vi "Garbagio-AB_BC_Chopper.vi"(9 "Portion of data":cluster{dbl, dbl}(slide)={0.75, 0.25} scale=0.0..1.0, 10 "Array of Clusters BC":cluster{dbl[], dbl[]}[](array[cluster]), 11 "Array of Clusters AB":cluster{dbl[], dbl[]}[](array[cluster])) -> (2 "Chopped AB thing":cluster{dbl[], dbl[]}, 3 "Chopped BC thing":cluster{dbl[], dbl[]})   [LabVIEW 2016]
uses:
  <vilib>/Analysis/2dsp.llb/Decimate (single shot, DBL).vi
  <vilib>/Analysis/NI_AALPro.lvlib
panel:
  in  "Decimate point":dbl=1e-10 format="%#_1f"
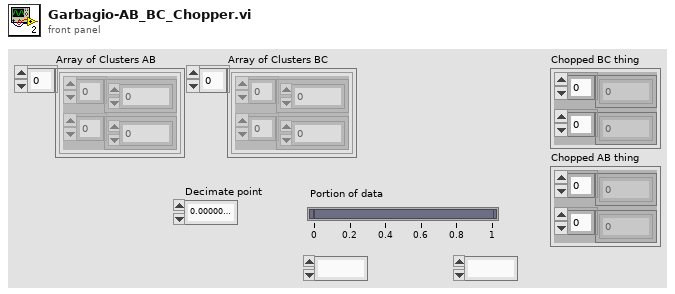
[diagram p1: front panel]
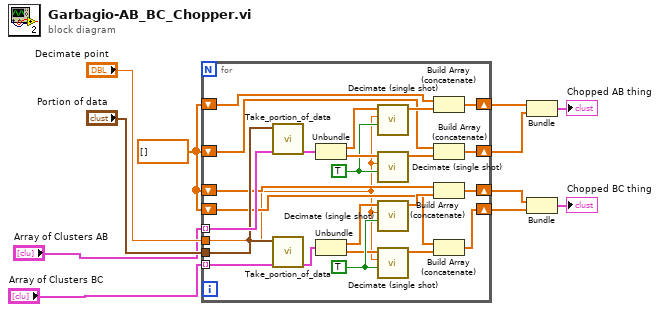
[diagram p0: block diagram]
diagram:
  w7 = dbl[] []
  n1 = for {
    tunnel: "Array of Clusters AB" -> [w35] mode=indexing
    tunnel: "Array of Clusters BC" -> [w18] mode=indexing
    tunnel: "Portion of data" -> [w17]
    tunnel: "Decimate point" -> [w12]
    shift-right: [w30] -> w9
    shift-left: w7 -> [w28]
    shift-right: [w26] -> w8
    shift-left: w7 -> [w25]
    shift-right: [w16] -> w6
    shift-left: w7 -> [w15]
    shift-right: [w14] -> w5
    shift-left: w7 -> [w13]
    w21 = TRUE ("averaging")
    w32 = TRUE ("averaging")
    n2 = call <userlib>:"Take_portion_of_data.vi"("input IV"=w35, "Slide"=w17) -> ("Output IV"=w31:cluster{dbl[], dbl[]})  [unwired: 5 in]
    n3 = call <userlib>:"Take_portion_of_data.vi"("input IV"=w18, "Slide"=w17) -> ("Output IV"=w22:cluster{dbl[], dbl[]})  [unwired: 5 in]
    n4 = Unbundle(w31) -> (w33:dbl[], w34:dbl[])
    n5 = Unbundle(w22) -> (w20:dbl[], w19:dbl[])
    n6 = call-poly <vilib>:"Decimate (single shot).vi"("averaging"=w32, "decimating factor"=w12, "X"=w33) -> ("Decimated Array"=w29:dbl[])  [unwired: 7 in, 1 out]
    n7 = call-poly <vilib>:"Decimate (single shot).vi"("averaging"=w32, "decimating factor"=w12, "X"=w34) -> ("Decimated Array"=w27:dbl[])  [unwired: 7 in, 1 out]
    n8 = call-poly <vilib>:"Decimate (single shot).vi"("averaging"=w21, "decimating factor"=w12, "X"=w20) -> ("Decimated Array"=w23:dbl[])  [unwired: 7 in, 1 out]
    n9 = call-poly <vilib>:"Decimate (single shot).vi"("averaging"=w21, "decimating factor"=w12, "X"=w19) -> ("Decimated Array"=w24:dbl[])  [unwired: 7 in, 1 out]
    n10 = Build Array (concatenate)(w28, w29) -> (w30:dbl[])
    n11 = Build Array (concatenate)(w25, w27) -> (w26:dbl[])
    n12 = Build Array (concatenate)(w15, w23) -> (w16:dbl[])
    n13 = Build Array (concatenate)(w13, w24) -> (w14:dbl[])
  }
  n14 = Bundle(w9, w8) -> (→"Chopped AB thing":cluster{dbl[], dbl[]})  [unwired: 1 in]
  n15 = Bundle(w6, w5) -> (→"Chopped BC thing":cluster{dbl[], dbl[]})  [unwired: 1 in]
